vi "ROI group-Generate ROI group image.vi"(8 "error in (no error)":errorcluster) -> (0 "error out":errorcluster, 1 "Group Name":string, 2 "Red & Green ROI group image cluster":T2, 3 "Image to display":T1)   [LabVIEW 2020]
uses:
  <vilib>/vision/Image Controls.llb/IMAQ Image.ctl
  Global variables/gl_Functional Imaging-Global variables.vi
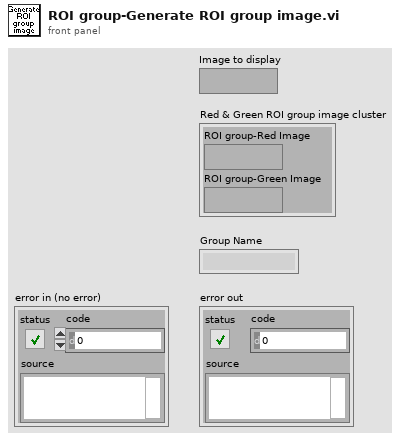
[diagram p1: front panel]
types:
  T1 = typedef "IMAQ Image.ctl" = refnum<image>
  T2 = cluster{"ROI group-Red Image":T1, "ROI group-Green Image":T1}
  T3 = typedef "Functional Imging UI Refs.ctl" = cluster{"Menu ref":refnum<k9>, "Image control":refnum<vi>, "VI ref":refnum<vi>, "XGrapher":refnum<vi>, "Smoothing":refnum<vi>, "POI Averaging":refnum<vi>, "Normalize":refnum<vi>, "POI data points in each trial":refnum<vi>, "Channel":refnum<vi>, "Experiment data folder path":refnum<vi>, "[ROI vis]":refnum<vi>, "[Groups] visbl":T4, "Group Name":refnum<vi>, "POI index":refnum<vi>, "Trial No.":refnum<vi>, "Intensity Zoom":refnum<vi>, "Trial Cursor Enabled":refnum<vi>, "Number of Trials (ind 1)":refnum<vi>, "Number of Trials (ind 2)":refnum<vi>, "MiniScans Available":refnum<vi>, "POI Available":refnum<vi>, "Defer graph updates":refnum<vi>, "Waveform selector":refnum<vi>, "#of selected POI":refnum<vi>, "#of selected MiniScans":refnum<vi>, "#of selected groups":refnum<vi>, "Max Z-Projection":refnum<vi>, "Z-Plane Selector":refnum<vi>, "Index of miniscan point to visualise":refnum<vi>, "ROI vis. mode":refnum<vi>, "Total # of points":refnum<vi>, "Index of group clicked on":refnum<vi>, "Pane 1":refnum<vi>, "Pane 2":refnum<vi>, "Pane 3":refnum<vi>, "Pane 4":refnum<vi>, "Pane 5":refnum<vi>, "Pane 6":refnum<vi>, "Deselect all ROI":refnum<vi>, "Deselect all groups":refnum<vi>}
  T4 = typedef "Groups array referecne.ctl" = refnum<vi>
  T5 = typedef "Group sel cluster.ctl" = cluster{"Group number":string, "Group Name":string, "Visibility":bool, "Highlight":bool}
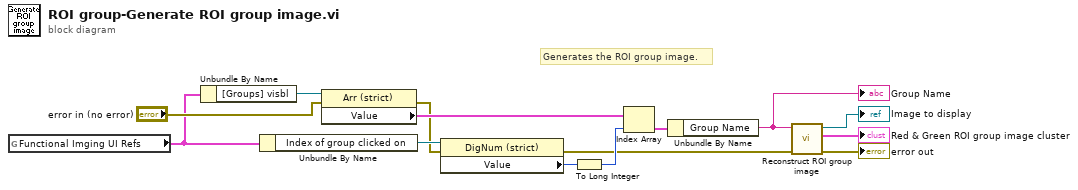
[diagram p0: block diagram]
diagram:
  # "Generates the ROI group image."
  n1 = global read "gl_Functional Imaging-Global variables.vi" "Functional Imging UI Refs"() -> (w5:T3)
  n2 = Unbundle By Name(w5) -> ("[Groups] visbl"=w8:T4)
  n3 = Unbundle By Name(w5) -> ("Index of group clicked on"=w13:refnum<vi>)
  n4 = property on="Property Node" class="Arr (strict)"(reference=w8, error in="error in (no error)") -> (error out=w6:errorcluster, "Value"=w10:T5[])  [unwired: 1 out]
  n5 = property on="Property Node" class="DigNum (strict)"(reference=w13, error in=w6) -> (error out=w2:errorcluster, "Value"=w14:i16)  [unwired: 1 out]
  n6 = To Long Integer(number=w14) -> (32bit integer=w12:i32)
  n7 = Index Array(array=w10, index=w12) -> (element=w11:T5)
  n8 = Unbundle By Name(w11) -> ("Group Name"=w1:string)
  "Group Name" <- w1
  n9 = call "Reconstruct ROI group image.vi"("error in"=w2, "Name of ROI group to search for"=w1) -> ("error out"=→"error out":errorcluster, "Red & Green ROI group image cluster"=→"Red & Green ROI group image cluster":T2, "Image to display"=→"Image to display":T1)  [unwired: 7 in]
